vi "Write StateManager.vi"(8 "error in (no error)":errorcluster, 10 "StateManager":refnum<class "StateManager.lvclass">, 11 "ICS in":refnum<class "ICS.lvclass">) -> (0 "error out":errorcluster, 3 "ICS out":refnum<class "ICS.lvclass">)   [LabVIEW 2018, in "ICS.lvclass"]
uses:
  ICS.lvclass
  StateManager/StateManager.lvclass
  ICS.lvclass/ICS.ctl
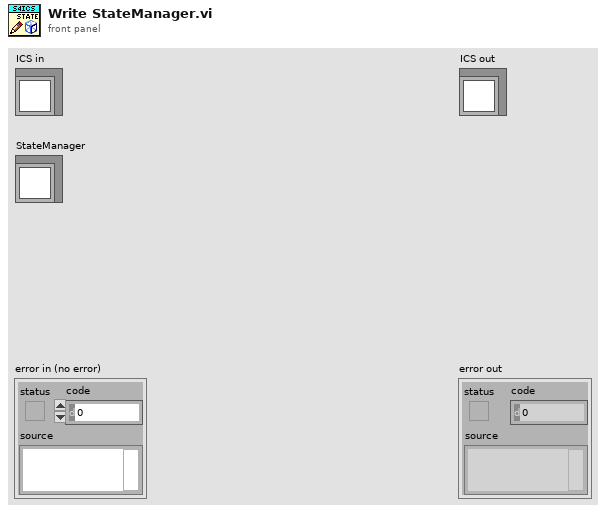
[diagram p1: front panel]
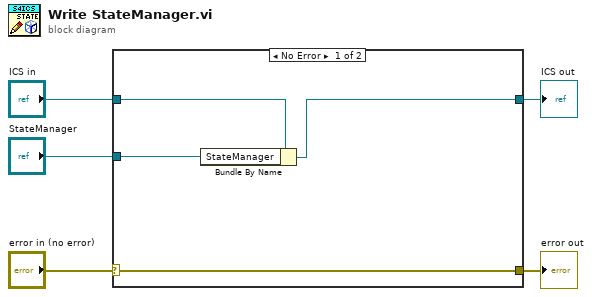
[diagram p0: block diagram]
diagram:
  n1 = case shown="No Error" "error in (no error)" {
    selector: "error in (no error)" -> [w9 w10]
    tunnel: [w9 w10] -> w4
    tunnel: [w6 w11] -> w2
    tunnel: "ICS in" -> [w8 w11]
    tunnel: "StateManager" -> [w7 _]
    frame No Error {
      n2 = Bundle By Name(cluster=w8, "StateManager"=w7) -> (w6:refnum<class "ICS.lvclass">)
    }
    frame Error {
    }
  }
  "error out" <- w4
  "ICS out" <- w2
